vi "DI Data.vi"(9 "Enum":enum16{"Write", "Read"}(ring), 11 "DI Data":bool[](array[boolean])) -> (3 "DI Data":bool[](array[boolean]))   [LabVIEW 2022 SP3]
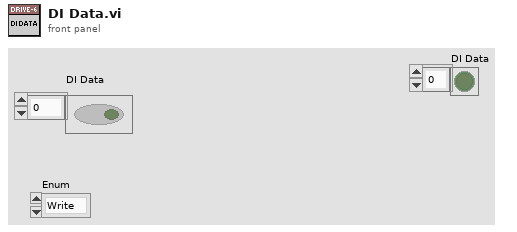
[diagram p1: front panel]
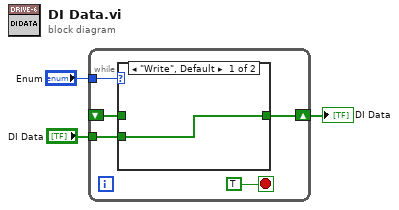
[diagram p0: block diagram]
diagram:
  n1 = while {
    tunnel: "Enum" -> [w7]
    tunnel: "DI Data" -> [w6]
    shift-right: [w5] -> w1
    shift-left: _ -> [w4]
    stop <- TRUE stop-if-true
    n2 = case shown="\"Write\", Default" w7 {
      tunnel: w6 -> [w9 _]
      tunnel: [w9 w10] -> w5
      tunnel: w4 -> [_ w10]
      frame "Write", Default {
      }
      frame "Read" {
      }
    }
  }
  "DI Data" <- w1
